vi "isotope_to_value.vi"(9 "MFT name":string, 10 "magnet string in":string) -> (2 "magnet value out":dbl)   [LabVIEW 2018]
doc: "Input is string.\nIf input string is an isotope name (as given in the magfieldtables) it is being conveted into a magnet value.\nIf string also has [+-*/] computation is performed"
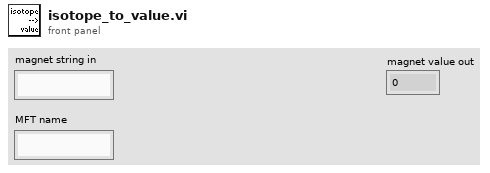
[diagram p1: front panel]
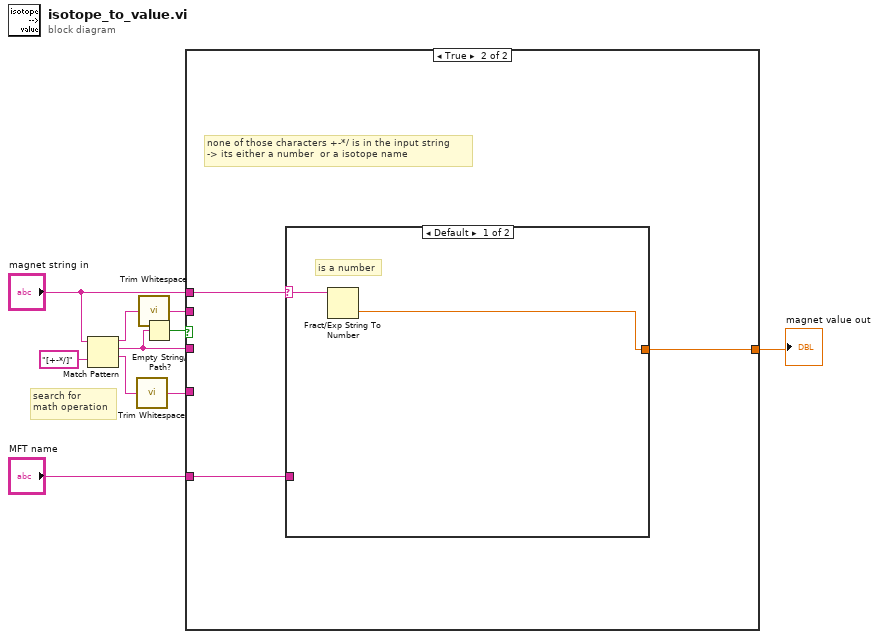
[diagram p0: block diagram]
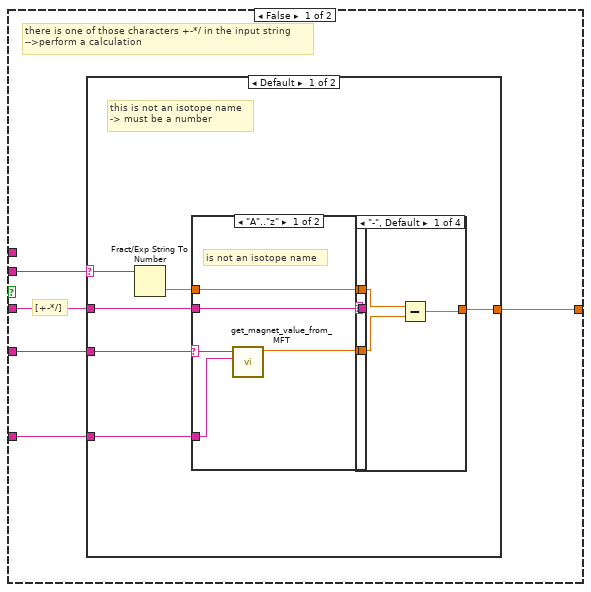
[diagram p2: hidden frame]
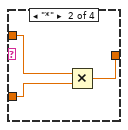
[diagram p3: hidden frame]
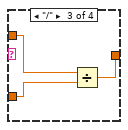
[diagram p4: hidden frame]
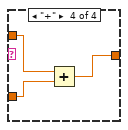
[diagram p5: hidden frame]
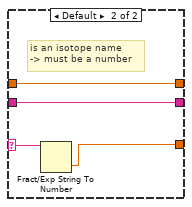
[diagram p6: hidden frame]
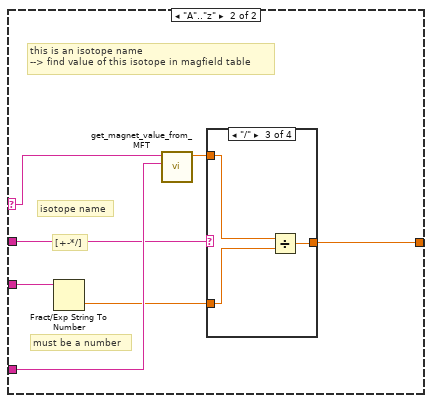
[diagram p7: hidden frame]
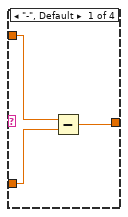
[diagram p8: hidden frame]
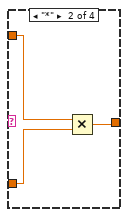
[diagram p9: hidden frame]
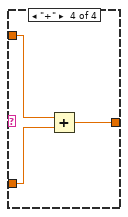
[diagram p10: hidden frame]
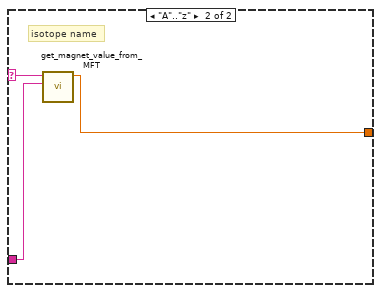
[diagram p11: hidden frame]
diagram:
  # "search for\nmath operation"
  n1 = Match Pattern(string="magnet string in", regular expression="[+-*/]") -> (before substring=w5:string, match substring=w2:string, after substring=w3:string)  [unwired: 1 in, 1 out]
  n2 = call <vilib>:"Trim Whitespace.vi"("string"=w3) -> ("trimmed string"=w4:string)  [unwired: 1 in]
  n3 = call <vilib>:"Trim Whitespace.vi"("string"=w5) -> ("trimmed string"=w6:string)  [unwired: 1 in]
  n4 = Empty String/Path?(string/path=w2) -> (empty?=w10:bool)
  n5 = case shown="True" w10 {
    tunnel: "magnet string in" -> [_ w67]
    tunnel: w6 -> [w15 _]
    tunnel: w4 -> [w14 _]
    tunnel: "MFT name" -> [w13 w66]
    tunnel: w2 -> [w12 _]
    tunnel: [w11 w65] -> w1
    frame False {
      # "[+-*/]"
      # "there is one of those characters +-*/ in the input string\n-->perform a calculation"
      n6 = case shown="Default" w15 {
        selector: w15 -> [w24 w50]
        tunnel: w14 -> [w23 w52]
        tunnel: w13 -> [w20 w51]
        tunnel: w12 -> [w21 w49]
        tunnel: [w16 w46] -> w11
        frame Default {
          # "this is not an isotope name\n-> must be a number"
          n7 = Fract/Exp String To Number(string=w24) -> (number=w22:dbl)  [unwired: 3 in, 1 out]
          n8 = case shown="\"A\"..\"z\"" w23 {
            selector: w23 -> [w41 w45]
            tunnel: w22 -> [w39 w44]
            tunnel: w21 -> [w37 w42]
            tunnel: w20 -> [w40 _]
            tunnel: [w39 w44] -> w19
            tunnel: [w38 w43] -> w18
            tunnel: [w37 w42] -> w17
            frame "A".."z" {
              # "is not an isotope name"
              n9 = call "get_magnet_value_from_MFT.vi"("MFT name"=w40, "isotope name"=w41) -> ("magnet value out"=w38:dbl)  [unwired: 9 in]
            }
            frame Default {
              # "is an isotope name\n-> must be a number"
              n10 = Fract/Exp String To Number(string=w45) -> (number=w43:dbl)  [unwired: 3 in, 1 out]
            }
          }
          n11 = case shown="\"-\", Default" w17 {
            tunnel: w19 -> [w27 w30 w33 w36]
            tunnel: w18 -> [w26 w29 w32 w35]
            tunnel: [w25 w28 w31 w34] -> w16
            frame "-", Default {
              n12 = Subtract(x=w27, y=w26) -> (x-y=w25:dbl)
            }
            frame "*" {
              n13 = Multiply(x=w30, y=w29) -> (x*y=w28:dbl)
            }
            frame "/" {
              n14 = Divide(x=w33, y=w32) -> (x/y=w31:dbl)
            }
            frame "+" {
              n15 = Add(x=w36, y=w35) -> (x+y=w34:dbl)
            }
          }
        }
        frame "A".."z" {
          # "[+-*/]"
          # "isotope name"
          # "must be a number"
          # "this is an isotope name\n--> find value of this isotope in magfield table"
          n16 = Fract/Exp String To Number(string=w52) -> (number=w47:dbl)  [unwired: 3 in, 1 out]
          n17 = call "get_magnet_value_from_MFT.vi"("MFT name"=w51, "isotope name"=w50) -> ("magnet value out"=w48:dbl)  [unwired: 9 in]
          n18 = case shown="\"/\"" w49 {
            tunnel: w48 -> [w55 w58 w61 w64]
            tunnel: w47 -> [w54 w57 w60 w63]
            tunnel: [w53 w56 w59 w62] -> w46
            frame "-", Default {
              n19 = Subtract(x=w55, y=w54) -> (x-y=w53:dbl)
            }
            frame "*" {
              n20 = Multiply(x=w58, y=w57) -> (x*y=w56:dbl)
            }
            frame "/" {
              n21 = Divide(x=w61, y=w60) -> (x/y=w59:dbl)
            }
            frame "+" {
              n22 = Add(x=w64, y=w63) -> (x+y=w62:dbl)
            }
          }
        }
      }
    }
    frame True {
      # "none of those characters +-*/ is in the input string\n-> its either a number  or a isotope name"
      n23 = case shown="Default" w67 {
        selector: w67 -> [w69 w72]
        tunnel: w66 -> [_ w71]
        tunnel: [w68 w70] -> w65
        frame Default {
          # "is a number"
          n24 = Fract/Exp String To Number(string=w69) -> (number=w68:dbl)  [unwired: 3 in, 1 out]
        }
        frame "A".."z" {
          # "isotope name"
          n25 = call "get_magnet_value_from_MFT.vi"("MFT name"=w71, "isotope name"=w72) -> ("magnet value out"=w70:dbl)  [unwired: 9 in]
        }
      }
    }
  }
  "magnet value out" <- w1
